vi "全局 水样时间.vi"() -> ()   [LabVIEW 2016, in "数据传输系统-04.lvlib"]
panel:
  in  "数据查表起始时间":T1
  in  "剖面数据时间":string
  in  "剖面多参数数据时间":string
  in  "水样数据索引":T2
  in  "选择发送的参数":string
  in  "小时数据时间":string
  in  "时间":string
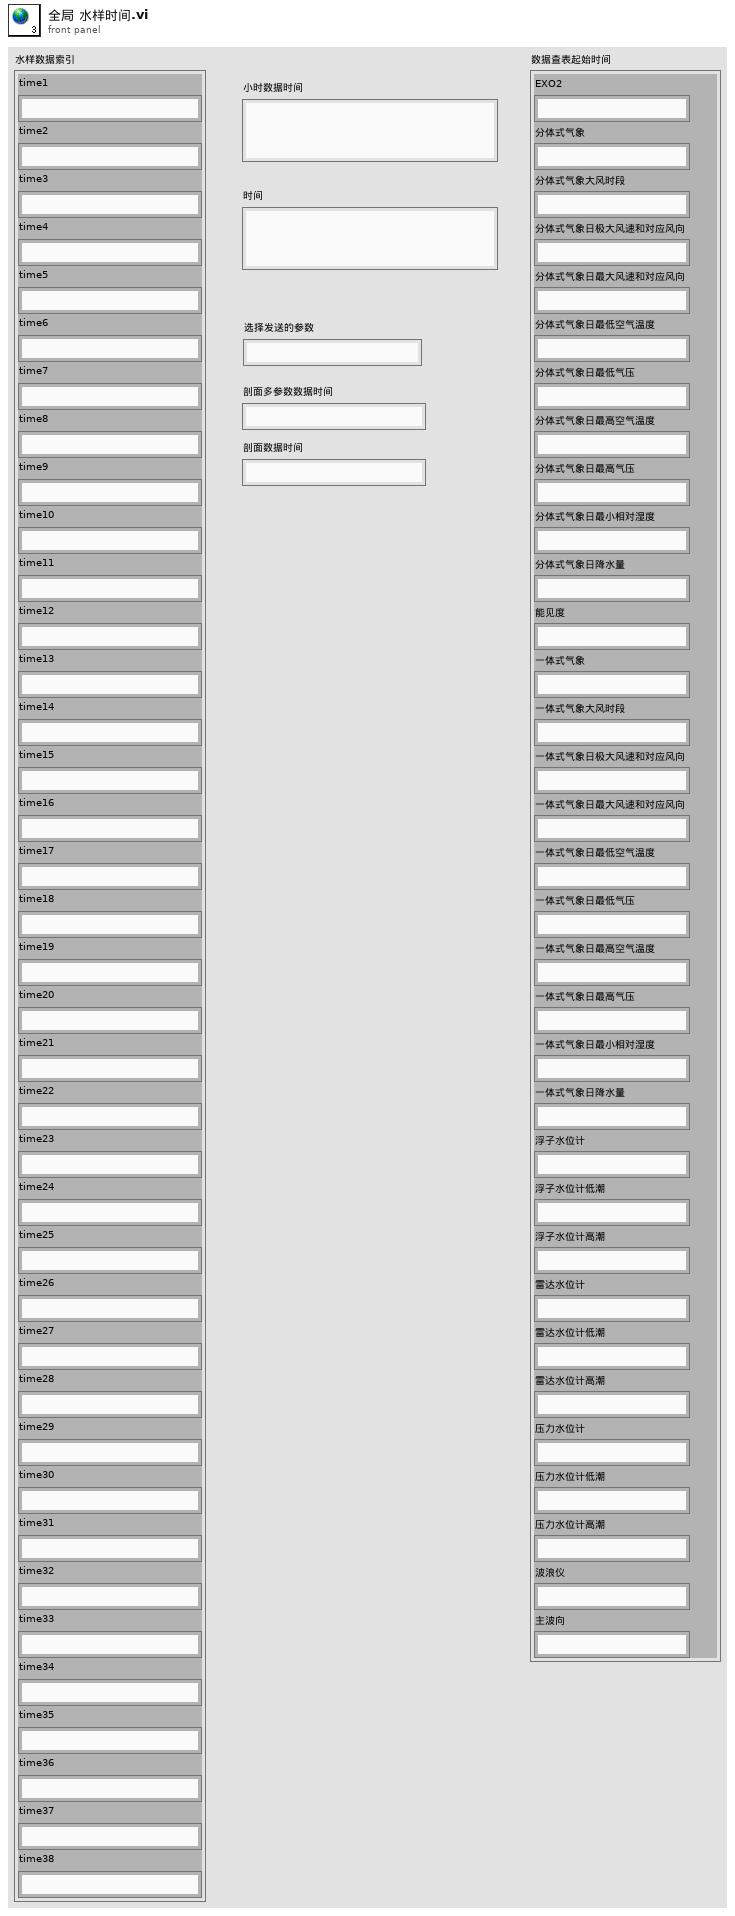
[diagram p1: front panel]
types:
  T1 = cluster{"EXO2":string, "分体式气象":string, "分体式气象大风时段":string, "分体式气象日极大风速和对应风向":string, "分体式气象日最大风速和对应风向":string, "分体式气象日最低空气温度":string, "分体式气象日最低气压":string, "分体式气象日最高空气温度":string, "分体式气象日最高气压":string, "分体式气象日最小相对湿度":string, "分体式气象日降水量":string, "能见度":string, "一体式气象":string, "一体式气象大风时段":string, "一体式气象日极大风速和对应风向":string, "一体式气象日最大风速和对应风向":string, "一体式气象日最低空气温度":string, "一体式气象日最低气压":string, "一体式气象日最高空气温度":string, "一体式气象日最高气压":string, "一体式气象日最小相对湿度":string, "一体式气象日降水量":string, "浮子水位计":string, "浮子水位计低潮":string, "浮子水位计高潮":string, "雷达水位计":string, "雷达水位计低潮":string, "雷达水位计高潮":string, "压力水位计":string, "压力水位计低潮":string, "压力水位计高潮":string, "波浪仪":string, "主波向":string}
  T2 = cluster{"time1":string, "time2":string, "time3":string, "time4":string, "time5":string, "time6":string, "time7":string, "time8":string, "time9":string, "time10":string, "time11":string, "time12":string, "time13":string, "time14":string, "time15":string, "time16":string, "time17":string, "time18":string, "time19":string, "time20":string, "time21":string, "time22":string, "time23":string, "time24":string, "time25":string, "time26":string, "time27":string, "time28":string, "time29":string, "time30":string, "time31":string, "time32":string, "time33":string, "time34":string, "time35":string, "time36":string, "time37":string, "time38":string}
diagram:
